vi "Get LTS Stage Max Velocity.vi"(8 "error in (no error)":errorcluster, 10 "Cluster in":T1, 11 "LTS Reference In":refnum<k24>) -> (0 "error out":errorcluster, 1 "VelocityMaximum":dbl, 2 "Cluster out":T1, 3 "LTS Reference Out":refnum<k24>)   [LabVIEW 2014]
uses:
  Controls/Translation Stage Cluster.ctl
  C:/Projects/Serial Sectioning OCT - TortoiseGIT/SerialSectOCT/Software/Thorlabs.MotionControl.Controls.dll
  Thorlabs.MotionControl.Controls.dll
  C:/Projects/Serial Sectioning OCT - TortoiseGIT/SerialSectOCT/Software/Thorlabs.MotionControl.IntegratedStepperMotorsCLI.dll
  Thorlabs.MotionControl.IntegratedStepperMotorsCLI.dll
  C:/Projects/Serial Sectioning OCT - TortoiseGIT/SerialSectOCT/Software/Thorlabs.MotionControl.GenericMotorCLI.dll
  Thorlabs.MotionControl.GenericMotorCLI.dll
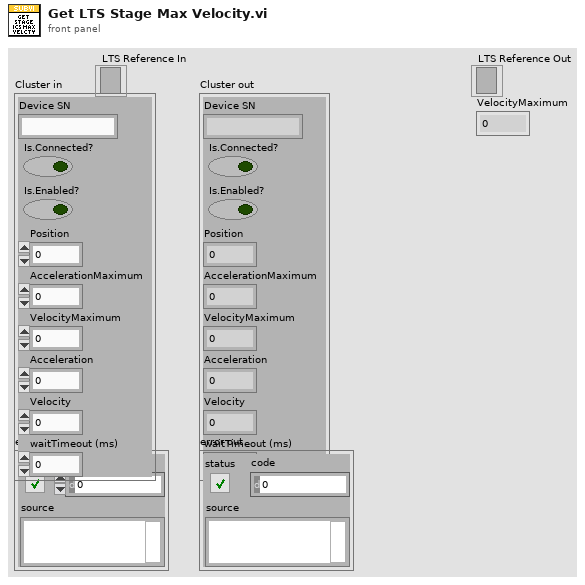
[diagram p1: front panel]
types:
  T1 = typedef "Translation Stage Cluster.ctl" = cluster{"Device SN":string, "Is.Connected?":bool, "Is.Enabled?":bool, "Position":dbl, "AccelerationMaximum":dbl, "VelocityMaximum":dbl, "Acceleration":dbl, "Velocity":dbl, "waitTimeout (ms)":i32}
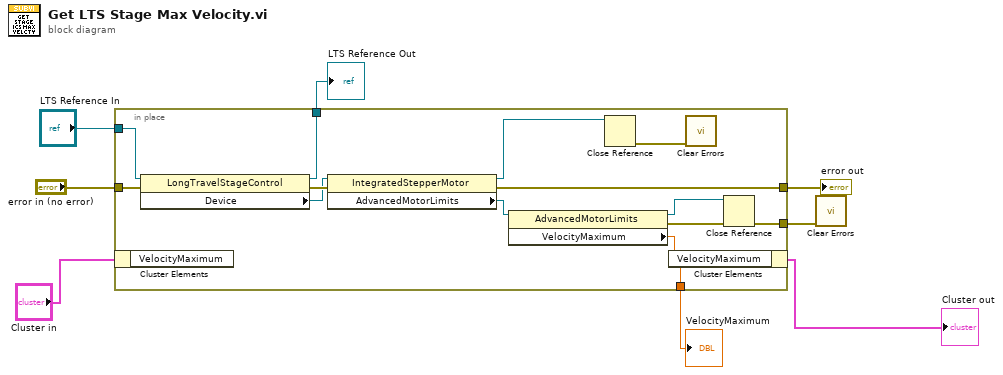
[diagram p0: block diagram]
diagram:
  n1 = in-place {
    in-place-border: [w21] -> w8
    in-place-border: [w9] -> w7
    in-place-border: [w17] -> w6
    in-place-border: "LTS Reference In" -> [w16]
    in-place-border: [w11] -> w4
    in-place-border: "error in (no error)" -> [w10]
    n2 = in-place-cluster #1("Cluster in") -> ()  [unwired: 1 out]
    n3 = property class="LongTravelStageControl"(reference=w16, error in=w10) -> (reference out=w11:refnum<k24>, error out=w15:errorcluster, "Device"=w12:refnum<k24>)
    n4 = property class="IntegratedStepperMotor"(reference=w12, error in=w15) -> (reference out=w14:refnum<k24>, error out=w17:errorcluster, "AdvancedMotorLimits"=w18:refnum<k24>)
    n5 = property class="AdvancedMotorLimits"(reference=w18) -> (reference out=w20:refnum<k24>, error out=w19:errorcluster, "VelocityMaximum"=w9:dbl)  [unwired: 1 in]
    n6 = Close Reference(reference=w14) -> (error out=w13:errorcluster)  [unwired: 1 in]
    n7 = in-place-cluster #1("VelocityMaximum"=w9) -> (→"Cluster out":T1)
    n8 = call <vilib>:"Clear Errors.vi"("error in (no error)"=w13) -> ()  [unwired: 5 in, 2 out]
    n9 = Close Reference(reference=w20, error in (no error)=w19) -> (error out=w21:errorcluster)
  }
  "error out" <- w6
  "LTS Reference Out" <- w4
  "VelocityMaximum" <- w7
  n10 = call <vilib>:"Clear Errors.vi"("error in (no error)"=w8) -> ()  [unwired: 5 in, 2 out]
